vi "Marker Line Style Read.vi"(4 "error in (no error)":errorcluster, 6 "Container State":T3, 7 "Display State In":T1) -> (0 "error out":errorcluster, 2 "Value":u8, 3 "Display State Out":T1)   [LabVIEW 2020, in "2D Error Bar.xctl"]
uses:
  <vilib>/Math Plots/2D Math Plots/2D Error Bar/2D Error Bar XCtrl/2D Error Bar.xctl
  <vilib>/_xctls/Container State.ctl
  <vilib>/Math Plots/2D Math Plots/2D Error Bar/2D Error Bar XCtrl/State.ctl
  <vilib>/Math Plots/2D Math Plots/2D Error Bar/2D Error Bar/2D Error Bar.lvclass
  e:/builds/penguin/labview/branches/2020/dev/dist/vi.lib/Math Plots/2D Math Plots/2D Plot/2D Plot/2D Plot.lvclass
  <vilib>/Math Plots/2D Math Plots/2D Plot/Action String/2DMathPlot Ctrl Act Queue.ctl
  <vilib>/Math Plots/2D Math Plots/2D Plot/Action String/2DMathPlot Ctrl Act Cluster.ctl
  <vilib>/Math Plots/2D Math Plots/2D Plot/Action String/2DMathPlot State Class.ctl
  <vilib>/Math Plots/2D Math Plots/2D Plot/2D Plot/2D Plot.lvclass
  <vilib>/_xctls/XControlSupport.lvlib
panel:
  # "Replace the Value Indicator below with an Indicator of desired type.\nDo not remove this Indicator or the others from the connector pane. \nDo not change the connector pane pattern.\nThe Value Indicator should always be the second terminal from top on the output side in the connector pane."
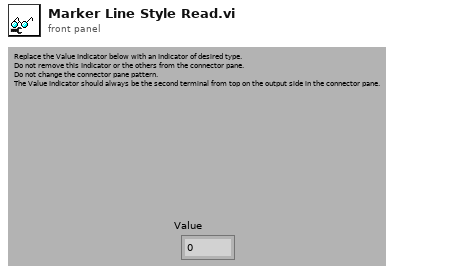
[diagram p1: front panel]
types:
  T1 = typedef "2D Error Bar.xctl/State.ctl" = cluster{"2D Error Bar.lvclass":refnum<class "2D Error Bar.lvclass">, "Control Ref Queue":T2, "Main Frame Color":u32, "Plot Legend Color":u32}
  T2 = typedef "2DMathPlot Ctrl Act Queue.ctl" = refnum<queue>
  T3 = typedef "XControlSupport.lvlib/Container State.ctl" = cluster{"Indicator?":bool, "Run Mode?":bool, " Refnum":refnum<vi>}
  T4 = typedef "2D Error Bar.lvclass/2D Error Bar Property Array.ctl" = T5[]
  T5 = typedef "2D Error Bar.lvclass/2D Error Bar Property.ctl" = cluster{"Marker Size":dbl, "Marker Line Style":u8, "Marker Line Width":u8, "Marker Color":u32, "Error Bar Interpolation":enum16{"Show Point", "Show Line", "Show Bar"}, "Error Mode":enum16{"Show Y Error", "Show X Error", "Show Both Error"}}
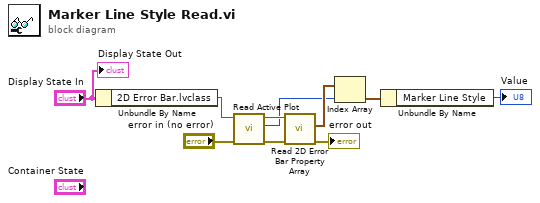
[diagram p0: block diagram]
diagram:
  n1 = Unbundle By Name("Display State In") -> ("2D Error Bar.lvclass"=w8:refnum<class "2D Error Bar.lvclass">)
  n2 = call <vilib>:"Read Active Plot.vi"("error in (no error)"="error in (no error)", "2D Plot.lvclass in"=w8) -> ("error out"=w5:errorcluster, "Active Plot"=w6:i32, "2D Plot.lvclass out"=w7:refnum<class "2D Error Bar.lvclass">)  [unwired: 7 out]
  n3 = call <vilib>:"Read 2D Error Bar Property Array.vi"("error in (no error)"=w5, "2D Error Bar.lvclass in"=w7) -> ("error out"=→"error out":errorcluster, "2D Error Bar Property Array"=w10:T4)  [unwired: 8 out]
  n4 = Index Array(array=w10, index=w6) -> (element=w9:T5)
  n5 = Unbundle By Name(w9) -> ("Marker Line Style"=→"Value":u8)
  "Display State Out" <- "Display State In"
